vi "Balance.vi"(2 "Balance Enabled":bool, 3 "Measured Angle":dbl=-1.6895785716878318, 4 "Right Motor Input":dbl=0.0009300018600037199, 5 "Left Motor Input":dbl=-0.0009300018600037199) -> (0 "Right Motor Output":dbl=0.0009300018600037199, 1 "Left Motor Output":dbl=-0.0009300018600037199)   [LabVIEW 2012]
uses:
  Robot Global Data.vi
panel:
  in  "angle threshold OLD":dbl=0.5
  in  "Distance to\n Balance  OLD":dbl=0.15
  in  "Speed to Balance OLD":dbl=1.0
  in  "Speed Low OLD":dbl=1.0
  in  "angle threshold":dbl=1.0
  in  "Distance to\n Balance":dbl=0.15
  in  "Speed to Balance":dbl=2.0
  in  "Speed Low":dbl=3.0
  out "Robot\nPitch Angle":dbl(knob)=-1.1556231756825557 scale=-20.0..20.0
  # "OLD"
  # "NEW"
  # "Feet/Second"
  # "Feet/Second"
  # "feet"
  # "feet"
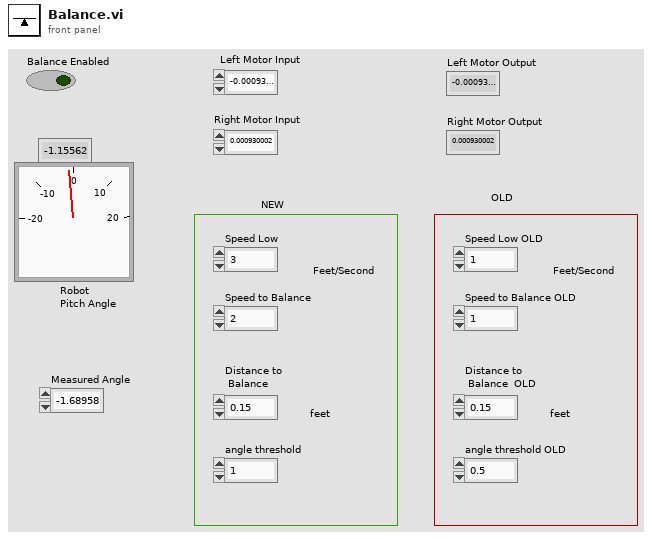
[diagram p1: front panel]
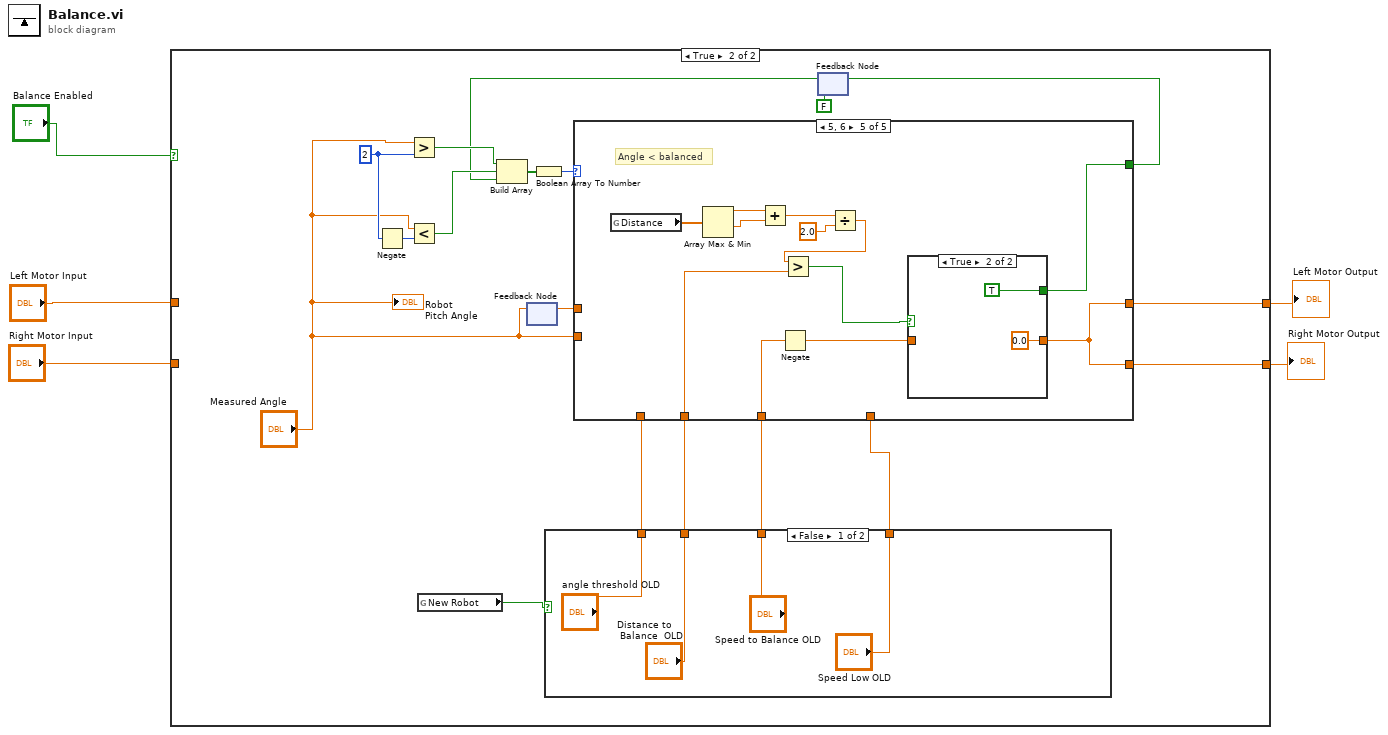
[diagram p0: block diagram]
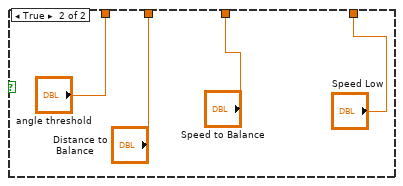
[diagram p3: hidden frame]
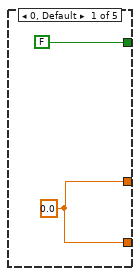
[diagram p4: hidden frame]
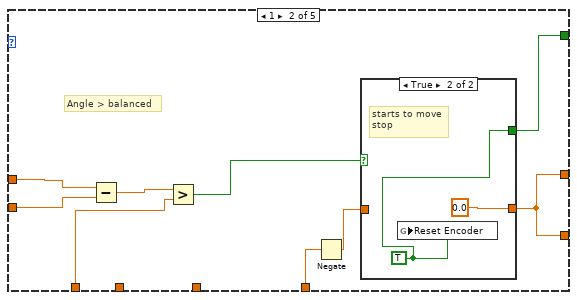
[diagram p5: hidden frame]
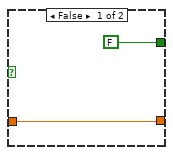
[diagram p6: hidden frame]
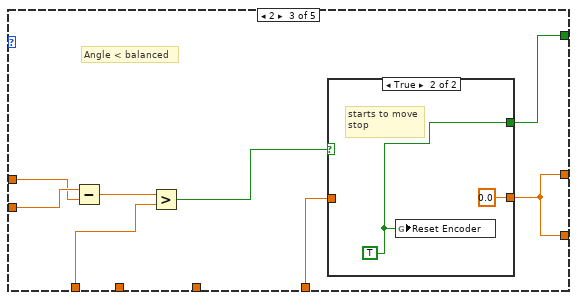
[diagram p7: hidden frame]
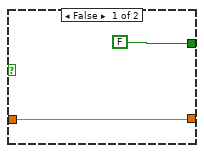
[diagram p8: hidden frame]
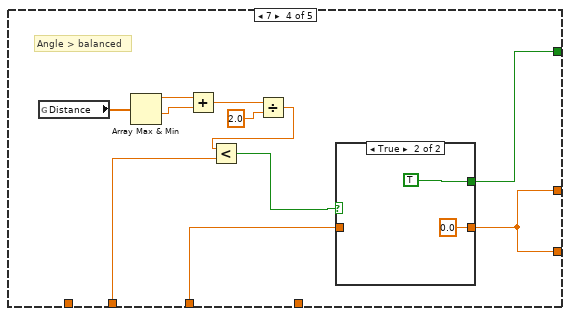
[diagram p9: hidden frame]
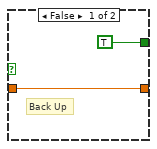
[diagram p10: hidden frame]
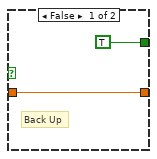
[diagram p11: hidden frame]
diagram:
  n1 = case shown="True" "Balance Enabled" {
    tunnel: [w7 w25] -> w5
    tunnel: "Right Motor Input" -> [w6 _]
    tunnel: "Left Motor Input" -> [w7 _]
    tunnel: [w6 w24] -> w2
    frame False {
    }
    frame True {
      w20 = 2
      n2 = Negate(x=w20) -> (-x=w19:i32)
      n3 = Greater?(x="Measured Angle", y=w20) -> (0:w22:bool)
      n4 = Less?(x="Measured Angle", y=w19) -> (x < y?=w21:bool)
      n5 = global read "Robot Global Data.vi" "New Robot"() -> (w12:bool)
      n6 = feedback #1() -> (w17:dbl)  [unwired: 1 in]
      n7 = feedback-in #1("Measured Angle") -> ()
      n8 = case shown="False" w12 {
        tunnel: ["Distance to\n Balance  OLD" "Distance to\n Balance"] -> w11
        tunnel: ["angle threshold OLD" "angle threshold"] -> w10
        tunnel: ["Speed to Balance OLD" "Speed to Balance"] -> w9
        tunnel: ["Speed Low OLD" "Speed Low"] -> w8
        frame False {
        }
        frame True {
        }
      }
      n9 = feedback #2(FALSE) -> (w14:bool)
      n10 = Build Array(w22, w21, w14) -> (w18:bool[])
      n11 = Boolean Array To Number(Boolean array=w18) -> (number=w23:u32)
      n12 = case shown="5, 6" w23 {
        tunnel: [w35 w39 w51 w64 w86] -> w25
        tunnel: [w35 w39 w51 w64 w86] -> w24
        tunnel: w8 -> [_ w41 w50 _ _]
        tunnel: "Measured Angle" -> [_ w42 w56 _ _]
        tunnel: w17 -> [_ w43 w55 _ _]
        tunnel: w9 -> [_ _ _ w62 w87]
        tunnel: w11 -> [_ _ _ w61 w83]
        tunnel: w10 -> [_ w40 w53 _ _]
        tunnel: [FALSE w36 w49 w63 w84] -> w15
        frame 0, Default {
          w35 = 0.0 ("Left Motor Input")
        }
        frame 1 {
          # "Angle > balanced"
          n13 = Subtract(x=w43, y=w42) -> (x-y=w44:dbl)
          n14 = Greater?(x=w44, y=w40) -> (0:w38:bool)
          n15 = Negate(x=w41) -> (-x=w37:dbl)
          n16 = case shown="True" w38 {
            tunnel: [w46 0.0 ("t")] -> w39
            tunnel: w37 -> [w46 _]
            tunnel: [FALSE w47] -> w36
            frame False {
            }
            frame True {
              w47 = TRUE
              # "starts to move\nstop"
              n17 = global write "Robot Global Data.vi" "Reset Encoder"(w47) -> ()
            }
          }
        }
        frame 2 {
          # "Angle < balanced"
          n18 = Subtract(x=w56, y=w55) -> (x-y=w54:dbl)
          n19 = Greater?(x=w54, y=w53) -> (0:w52:bool)
          n20 = case shown="True" w52 {
            tunnel: [w58 0.0 ("t")] -> w51
            tunnel: w50 -> [w58 _]
            tunnel: [FALSE w59] -> w49
            frame False {
            }
            frame True {
              w59 = TRUE
              # "starts to move\nstop"
              n21 = global write "Robot Global Data.vi" "Reset Encoder"(w59) -> ()
            }
          }
        }
        frame 7 {
          # "Angle > balanced"
          n22 = global read "Robot Global Data.vi" "Distance"() -> (w70:dbl[])
          n23 = Array Max & Min(array=w70) -> (max value=w69:dbl, min value=w68:dbl)  [unwired: 2 out]
          n24 = Add(x=w69, y=w68) -> (x+y=w67:dbl)
          n25 = Divide(x=w67, y=2.0) -> (x/y=w66:dbl)
          n26 = Less?(x=w66, y=w61) -> (x < y?=w71:bool)
          n27 = case shown="True" w71 {
            tunnel: [w73 0.0] -> w64
            tunnel: w62 -> [w73 _]
            tunnel: [TRUE TRUE] -> w63
            frame False {
              # "Back Up"
            }
            frame True {
            }
          }
        }
        frame 5, 6 {
          # "Angle < balanced"
          n28 = global read "Robot Global Data.vi" "Distance"() -> (w81:dbl[])
          n29 = Array Max & Min(array=w81) -> (max value=w80:dbl, min value=w79:dbl)  [unwired: 2 out]
          n30 = Add(x=w80, y=w79) -> (x+y=w78:dbl)
          n31 = Negate(x=w87) -> (-x=w85:dbl)
          n32 = Divide(x=w78, y=2.0) -> (x/y=w77:dbl)
          n33 = Greater?(x=w77, y=w83) -> (0:w82:bool)
          n34 = case shown="True" w82 {
            tunnel: [w89 0.0] -> w86
            tunnel: w85 -> [w89 _]
            tunnel: [TRUE TRUE] -> w84
            frame False {
              # "Back Up"
            }
            frame True {
            }
          }
        }
      }
      n35 = feedback-in #2(w15) -> ()
      "Robot\nPitch Angle" <- "Measured Angle"
    }
  }
  "Left Motor Output" <- w5
  "Right Motor Output" <- w2
